vi "12.2 Clusters to plot Data Graphs and Charts.vi"() -> ()   [LabVIEW 2019]
panel:
  out "XY Graph":cluster{dbl[], dbl[]}(graph)
  out "Graph":dbl[][](graph)
  out "Chart":cluster{dbl, dbl}(graph)
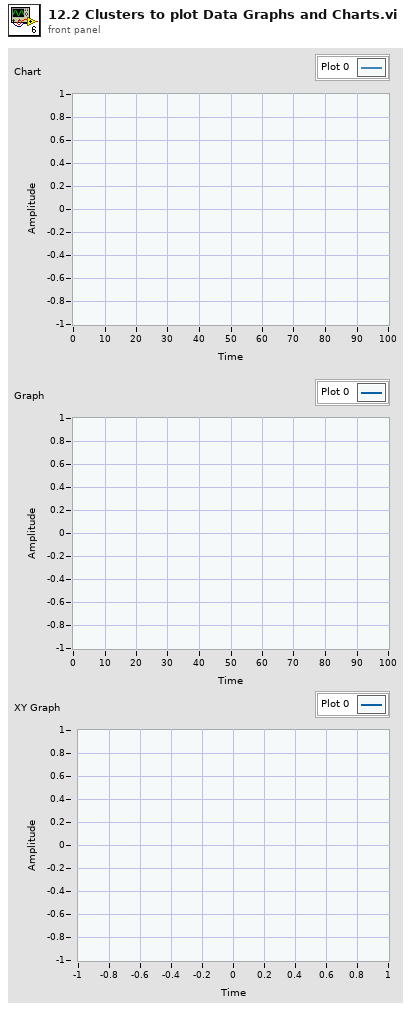
[diagram p1: front panel]
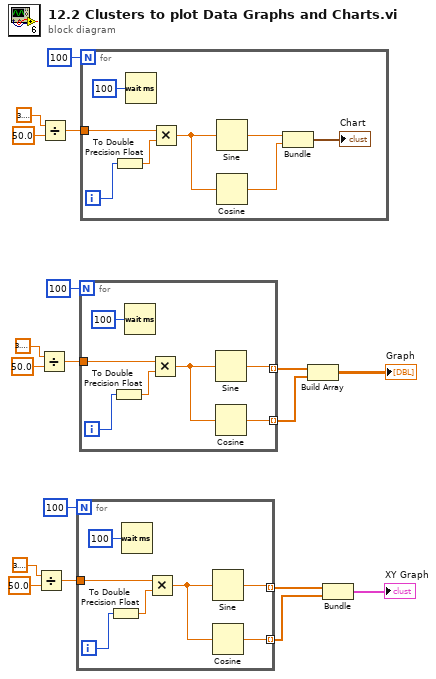
[diagram p0: block diagram]
diagram:
  n1 = Divide(x=3.141592653589793, y=50.0) -> (x/y=w4:dbl)
  n2 = Divide(x=3.141592653589793, y=50.0) -> (x/y=w14:dbl)
  n3 = Divide(x=3.141592653589793, y=50.0) -> (x/y=w15:dbl)
  n4 = for {
    N: 100 -> [_]
    tunnel: w4 -> [w22]
    tunnel: [w20] -> w3 mode=indexing
    tunnel: [w19] -> w2 mode=indexing
    i -> [w24]
    n5 = To Double Precision Float(number=w24) -> (double precision float=w23:dbl)
    n6 = Wait (ms)(milliseconds to wait=u32 100) -> ()  [unwired: 1 out]
    n7 = Multiply(x=w22, y=w23) -> (x*y=w21:dbl)
    n8 = Sine(x=w21) -> (sin(x)=w20:dbl)
    n9 = Cosine(x=w21) -> (cos(x)=w19:dbl)
  }
  n10 = for {
    N: 100 -> [_]
    tunnel: w14 -> [w29]
    tunnel: [w27] -> w10 mode=indexing
    tunnel: [w26] -> w9 mode=indexing
    i -> [w31]
    n11 = To Double Precision Float(number=w31) -> (double precision float=w30:dbl)
    n12 = Wait (ms)(milliseconds to wait=u32 100) -> ()  [unwired: 1 out]
    n13 = Multiply(x=w29, y=w30) -> (x*y=w28:dbl)
    n14 = Sine(x=w28) -> (sin(x)=w27:dbl)
    n15 = Cosine(x=w28) -> (cos(x)=w26:dbl)
  }
  n16 = for {
    N: 100 -> [_]
    tunnel: w15 -> [w37]
    i -> [w39]
    n17 = To Double Precision Float(number=w39) -> (double precision float=w38:dbl)
    n18 = Wait (ms)(milliseconds to wait=u32 100) -> ()  [unwired: 1 out]
    n19 = Multiply(x=w37, y=w38) -> (x*y=w36:dbl)
    n20 = Sine(x=w36) -> (sin(x)=w35:dbl)
    n21 = Cosine(x=w36) -> (cos(x)=w34:dbl)
    n22 = Bundle "Bundle"(w35, w34) -> (→"Chart":cluster{dbl, dbl})  [unwired: 1 in]
  }
  n23 = Build Array "Build Array"(w10, w9) -> (→"Graph":dbl[][])
  n24 = Bundle "Bundle"(w3, w2) -> (→"XY Graph":cluster{dbl[], dbl[]})  [unwired: 1 in]
